vi "configUI.vi"() -> ()   [LabVIEW 2017, in "AppStateMachine editor node.lvclass"]
doc: "All child modules share this same UI. The UI allows for the configuration of Channels, Parameters, and Error Handling."
uses:
  AppStateMachine editor node.lvclass
  <vilib>/NI/Configuration Framework/Node/NodeRef.ctl
  <vilib>/NI/Configuration Framework/Node/NISE_CEF_Node.lvclass
  <vilib>/NI/AMC/Message Queue.ctl
  <vilib>/NI/AMC/Message.ctl
  <vilib>/NI/Tools/Keyed Array/KeyedArray.ctl
  <vilib>/NI/Configuration Framework/Node/UserEventRef.ctl
  <vilib>/NI/Configuration Framework/Controls/EventCluster.ctl
  <vilib>/NI/DCAF/Tag Editor Core/control module/configuration/error classification setting.ctl
  <vilib>/NI/Tag Bus Module Framework/runtime/error classification.ctl
  <vilib>/NI/Configuration Framework/Node/RefreshUIEvent.ctl
  <vilib>/NI/Configuration Framework/Node/CacheState.ctl
  <vilib>/NI/Configuration Framework/Node/StopEvent.ctl
  <vilib>/NI/Configuration Framework/Node/NodeChangeEvent.ctl
  <vilib>/NI/DCAF/Tag Editor Core/Table API/Available Tag Menu/channel action event.ctl
  <vilib>/NI/DCAF/Tag Editor Core/Table API/Available Tag Menu/dialog output action.ctl
  <vilib>/NI/Tag Bus Module Framework/channel/TBM channel.lvclass
  <vilib>/NI/Tag Bus/tag/tag descriptor.lvclass
  <vilib>/NI/DCAF/Tag Editor Core/Table API/Table Manager/Call Back Ref Type Def.ctl
  <vilib>/NI/DCAF/Tag Editor Core/Configuration Editor/Classes/Engine Parent/Engine Parent Editor Node.lvclass
  <vilib>/NI/DCAF/Tag Editor Core/Configuration Editor/Classes/Module editor node/module editor node.lvclass
  C:/Program Files (x86)/National Instruments/LabVIEW 2017/vi.lib/NI/Configuration Framework/serializable node/NISE_CEF_serializable node.lvclass
  <vilib>/NI/DCAF/Tag Editor Core/Table API/Table Manager/references.ctl
  <vilib>/NI/DCAF/Tag Editor Core/Table API/Table Manager/Menu Definition.ctl
  <vilib>/NI/DCAF/Tag Editor Core/Table API/Table Manager/Menu Options.ctl
  <vilib>/NI/DCAF/Tag Editor Core/control module/configuration/control module configuration.lvclass
  C:/Program Files (x86)/National Instruments/LabVIEW 2017/vi.lib/NI/Configuration Framework/serializable configuration/NISE_CEF_serializable configuration.lvclass
  module/configuration/AppStateMachine configuration.lvclass
  C:/Program Files (x86)/National Instruments/LabVIEW 2017/vi.lib/NI/DCAF/Tag Editor Core/control module/configuration/control module configuration.lvclass
  C:/Program Files (x86)/National Instruments/LabVIEW 2017/vi.lib/NI/Tag Bus Module Framework/module configuration/TBM module configuration.lvclass
  C:/Program Files (x86)/National Instruments/LabVIEW 2017/vi.lib/NI/DCAF/Tag Editor Core/control module/editor node/control module editor.lvclass
  C:/Program Files (x86)/National Instruments/LabVIEW 2017/vi.lib/NI/DCAF/Tag Editor Core/Configuration Editor/Classes/Module editor node/module editor node.lvclass
  module/configuration/AppStateMachine configuration.lvclass/AppStateMachine configuration.ctl
  <vilib>/NI/DCAF/Tag Editor Core/control module/configuration/control module configuration.lvclass/control module configuration.ctl
  <vilib>/NI/Configuration Framework/serializable configuration/NISE_CEF_serializable configuration.lvclass/NISE_CEF_serializable configuration.ctl
  <vilib>/NI/Tag Bus Module Framework/channel/channel classification.ctl
  module/configuration/Read PrechargeTimeout.vi
  module/configuration/Read SynchronizeTimeout.vi
  module/configuration/Read DCLinkSteadyStateTimeout.vi
  module/configuration/Read PrechargeLevel.vi
  module/configuration/Read DCLinkSteadyState.vi
  module/configuration/Write PrechargeTimeout.vi
  module/configuration/Write SynchronizeTimeout.vi
  module/configuration/Write DCLinkSteadyStateTimeout.vi
  module/configuration/Write PrechargeLevel.vi
  module/configuration/Write DCLinkSteadyState.vi
  <vilib>/NI/DCAF/Tag Editor Core/control module/configuration/Write error classifications.vi
  <vilib>/NI/Tag Bus Module Framework/module configuration/TBM module configuration.lvclass
  <vilib>/NI/DCAF/Tag Editor Core/Configuration Editor/Classes/Module editor node/Read Module Configuration.vi
  <vilib>/NI/DCAF/Tag Editor Core/control module/editor node/read fixed channel configuration.vi
  <vilib>/NI/DCAF/Tag Editor Core/Configuration Editor/Classes/Module editor node/Write Module Configuration.vi
  <vilib>/Utility/LVClass/Get LV Class Name.vi
  <vilib>/NI/Configuration Framework/error generator/NISE_error generator.vi
  <vilib>/NI/Configuration Framework/serializable configuration/NISE_CEF_serializable configuration.lvclass
  <vilib>/NI/DCAF/Tag Editor Core/Table API/Listbox/Multi Column Listbox.lvclass
  <vilib>/NI/Configuration Framework/NISE_CEF_TreeControl.lvlib
  <vilib>/NI/DCAF/Tag Editor Core/Table API/Table Manager.lvlib
  <vilib>/NI/DCAF UI Toolkit/Controls/DCAF UI Elements.lvlib
  <vilib>/NI/Tools/Keyed Array/Tools_KeyedArray.lvlib
  <vilib>/NI/AMC/AMC.lvlib
  <vilib>/NI/DCAF/Tag Editor Core/Table API/Table Manager/Table Manager.lvclass
  <vilib>/NI/DCAF/Tag Editor Core/control module/editor node/control module editor.lvclass
  <vilib>/NI/Tag Bus Module Framework/runtime/TBM module execution interface.lvclass
panel:
  in  "Enum":i32
  in  "user event out":refnum<user-event>
  in  "Top Level Tab Control":T1(tab)
  in  "DCLinkSteadyState":dbl caption="DCLink Steady State (V)"
  in  "PrechargeLevel":dbl caption="Precharge Level (V)"
  in  "DCLinkSteadyStateTimeout":u32 caption="DCLink Steady State Timeout (ms)"
  in  "SynchronizeTimeout":u32 caption="Synchronize Timeout (ms)"
  in  "PrechargeTimeout":u32 caption="Precharge Timeout (ms)"
  in  "Channels Listbox":i32(listbox)
  in  "mapall":bool
  in  "mapwriters":bool
  in  "Parameters Listbox":i32(listbox)
  in  "error classifications":T2[](array[typedef])
  in  "node change":T4
  in  "stop event":T5
  in  "cache state":T6
  in  "refresh UI":T7
  in  "user event":T8
  in  "main queue":T9
  in  "node ref":T10
  # "(Single-Click to Edit)"
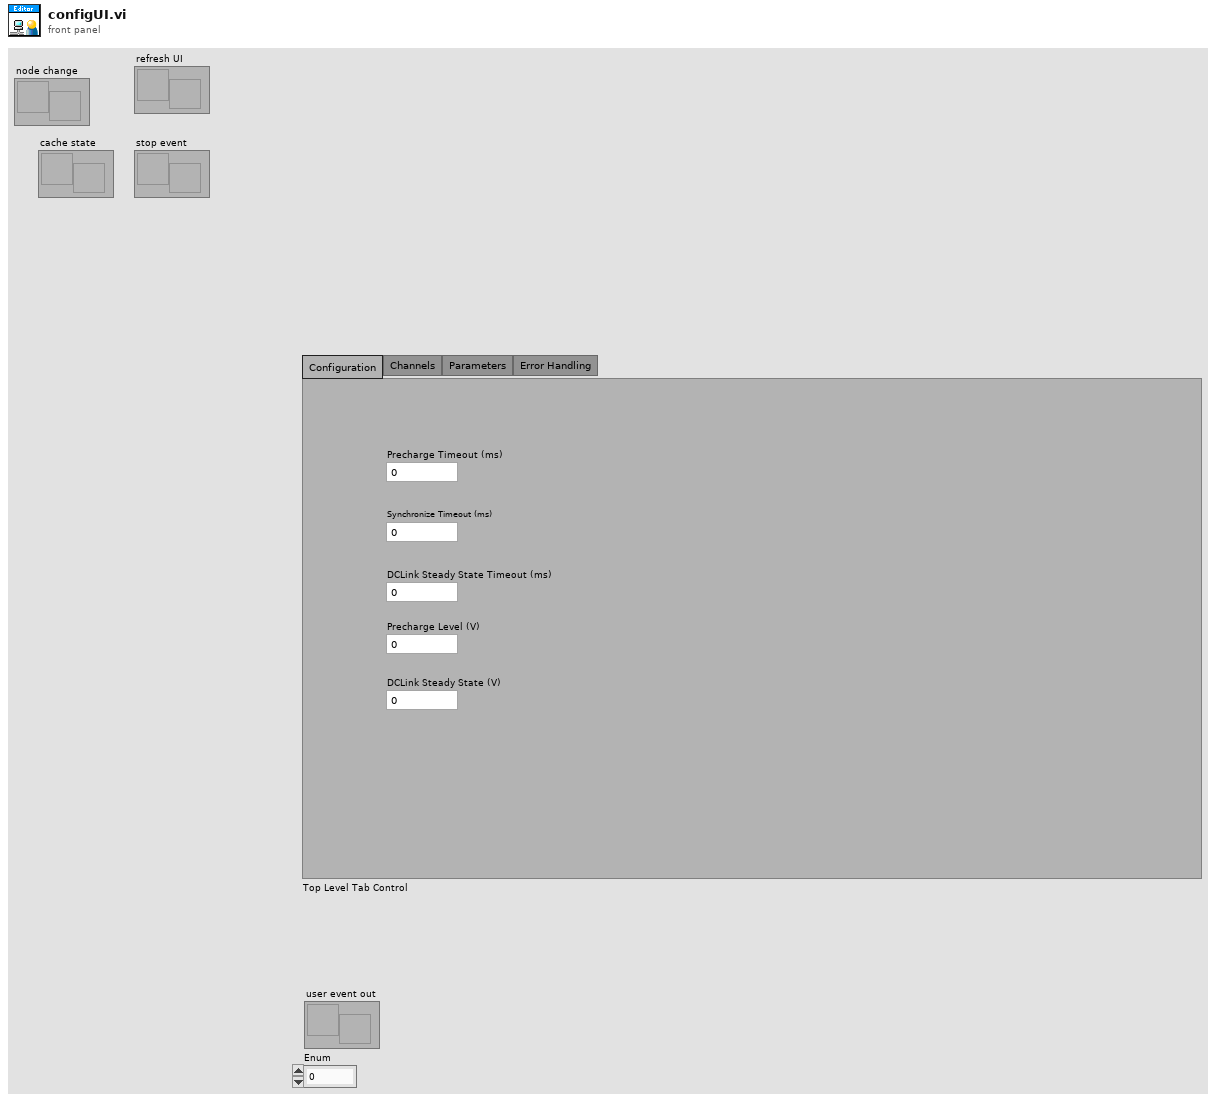
[diagram p1: front panel]
types:
  T1 = enum32{"Configuration", "Channels", "Parameters", "Error Handling"}
  T2 = typedef "control module configuration.lvclass/error classification setting.ctl" = cluster{"code":i32, "error classification":T3}
  T3 = typedef "TBM module execution interface.lvclass/error classification.ctl" = enum16{"unknown", "none", "trivial", "recoverable", "critical"}
  T4 = typedef "NISE_CEF_Node.lvclass/NodeChangeEvent.ctl" = refnum<user-event>
  T5 = typedef "NISE_CEF_Node.lvclass/StopEvent.ctl" = refnum<user-event>
  T6 = typedef "NISE_CEF_Node.lvclass/CacheState.ctl" = refnum<user-event>
  T7 = typedef "NISE_CEF_Node.lvclass/RefreshUIEvent.ctl" = refnum<user-event>
  T8 = typedef "NISE_CEF_Node.lvclass/UserEventRef.ctl" = refnum<user-event>
  T9 = typedef "AMC.lvlib/Message Queue.ctl" = refnum<queue>
  T10 = typedef "NISE_CEF_Node.lvclass/NodeRef.ctl" = refnum<data-value>
  T11 = typedef "Table Manager.lvlib/Table Manager.lvclass/Menu Definition.ctl" = cluster{"Menu Name":string, "Menu Options":T12}
  T12 = typedef "Table Manager.lvlib/Table Manager.lvclass/Menu Options.ctl" = enum16{"Always Show", "Show When Used", "Show When Empty"}
  T13 = typedef "Table Manager.lvlib/Table Manager.lvclass/references.ctl" = cluster{"stop event":T5, "refresh UI":T7, "cache state":T6, "node change":T4, "user event out":refnum<user-event>, "main queue":T9, "user event":T8}
  T14 = typedef "Table Manager.lvlib/Column.lvclass/Column Descriptor.ctl" = cluster{"name":string, "caption":string, "Column Type":T15, "Params":string, "AutoSizeMode":i32, "FillWeight":sgl, "MinWidth":u32, "tooltip":string, "Enum Reference":refnum<vi>, "Channel suffix":string, "Read Only":bool, "Call Back VI":T16, "DT Dependency":i32, "name dependency":i32, "data type":T17, "Custom Column":refnum<class "Column.lvclass">}
  T15 = typedef "Table Manager.lvlib/Column.lvclass/Column Type.ctl" = enum16{"String", "Mapping", "Enum", "Custom"}
  T16 = typedef "Table Manager.lvlib/Table Manager.lvclass/Call Back Ref Type Def.ctl" = refnum<vi>
  T17 = typedef "tag bus.lvlib/tag descriptor.lvclass/Data Type.ctl" = enum16{"Double", "Single", "I64", "I32", "I16", "I8", "U64", "U32", "U16", "U8", "Boolean", "String", "Array of Double", "Array of Single", "Array of I64", "Array of I32", "Array of I16", "Array of I8", "Array of U64", "Array of U32", "Array of U16", "Array of U8", "Array of Boolean", "Array of String"}
  T18 = typedef "Table Manager.lvlib/Table Manager.lvclass/object ref.ctl" = cluster{"engine":refnum<data-value>, "Node Ref":refnum<data-value>}
  T19 = typedef "Table Manager.lvlib/Table Manager.lvclass/Table Events.ctl" = cluster{"Menu Selection":refnum<user-event>}
  T20 = typedef "NISE_CEF_TreeControl.lvlib/EventCluster.ctl" = cluster{"command":string, "data":string}
  T21 = typedef "TBM channel.lvclass/channel classification.ctl" = enum16{"input data", "output data", "processing parameter", "processing result"}
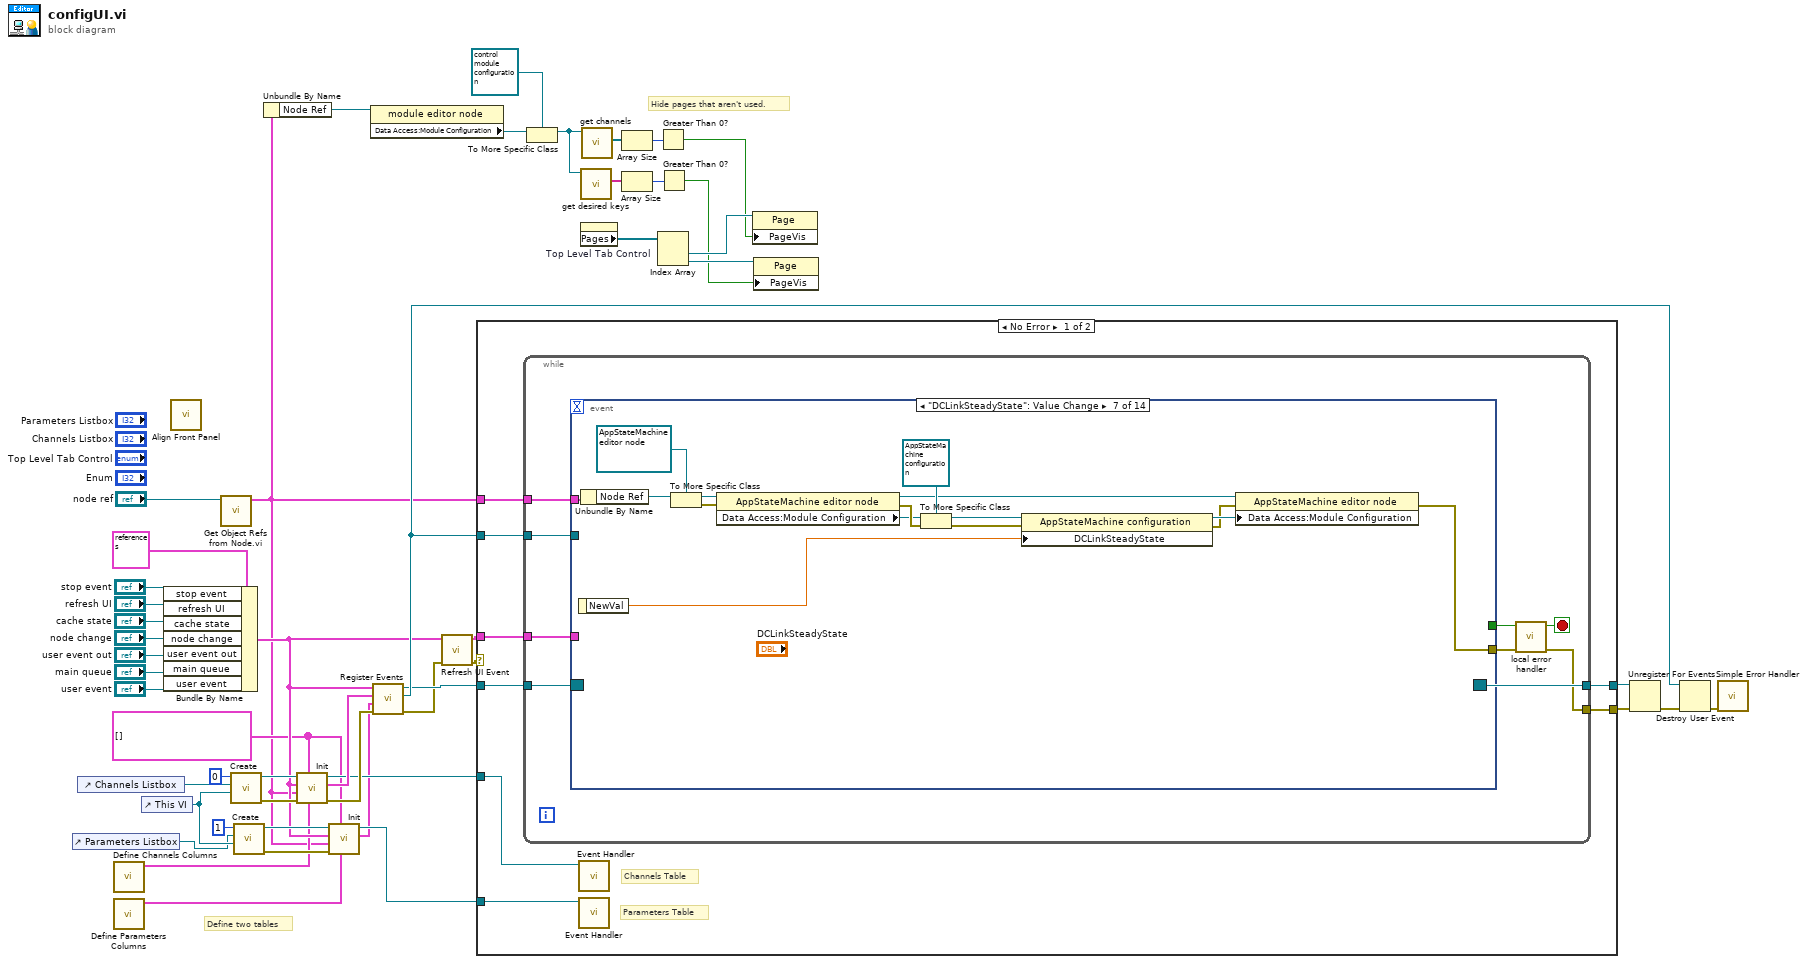
[diagram p0: block diagram]
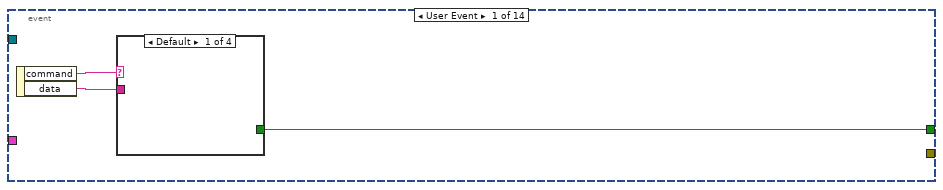
[diagram p2: hidden frame]
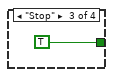
[diagram p4: hidden frame]
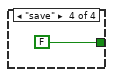
[diagram p5: hidden frame]
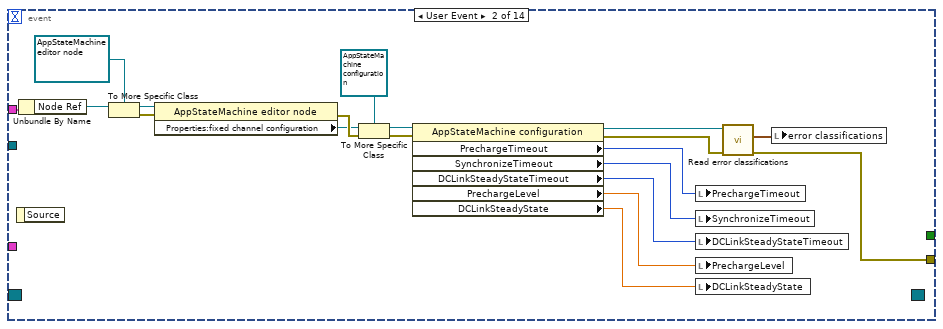
[diagram p6: hidden frame]
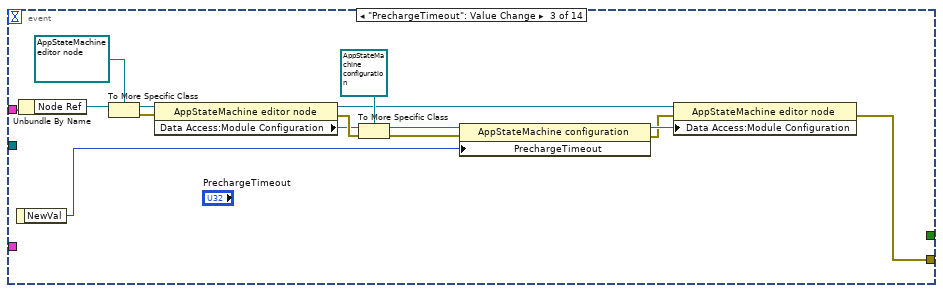
[diagram p7: hidden frame]
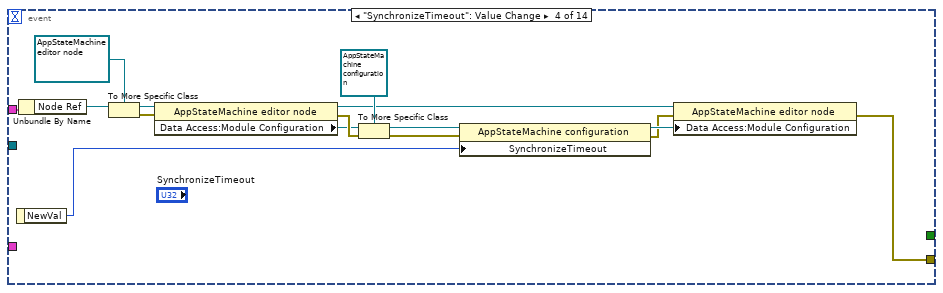
[diagram p8: hidden frame]
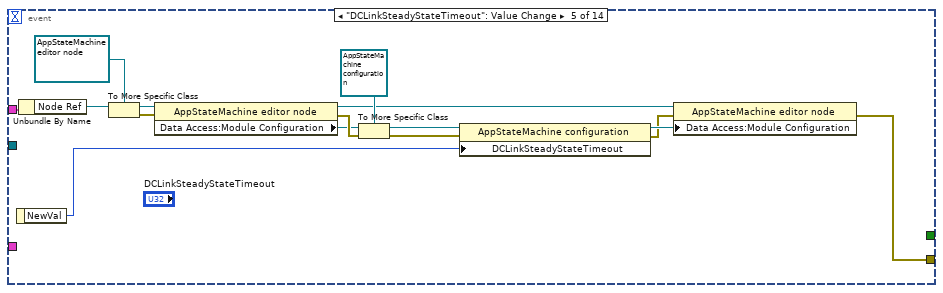
[diagram p9: hidden frame]
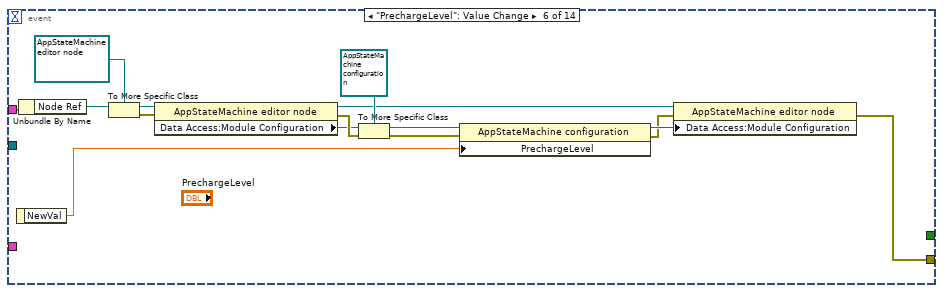
[diagram p10: hidden frame]
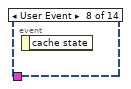
[diagram p11: hidden frame]
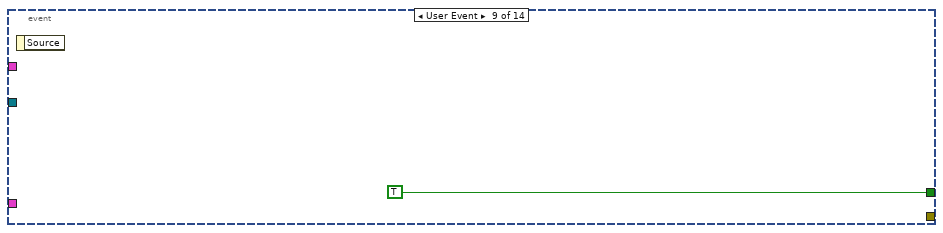
[diagram p12: hidden frame]
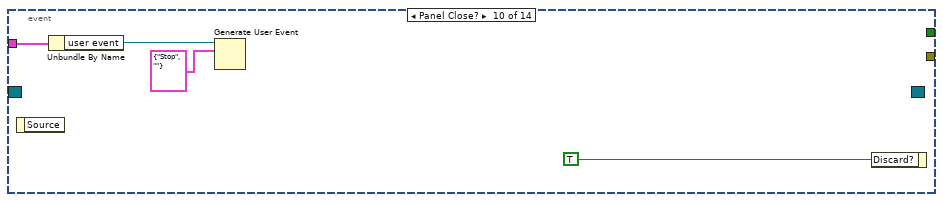
[diagram p13: hidden frame]
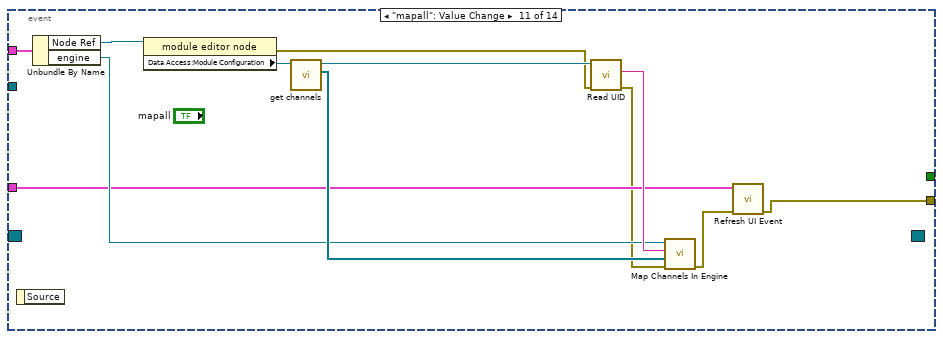
[diagram p14: hidden frame]
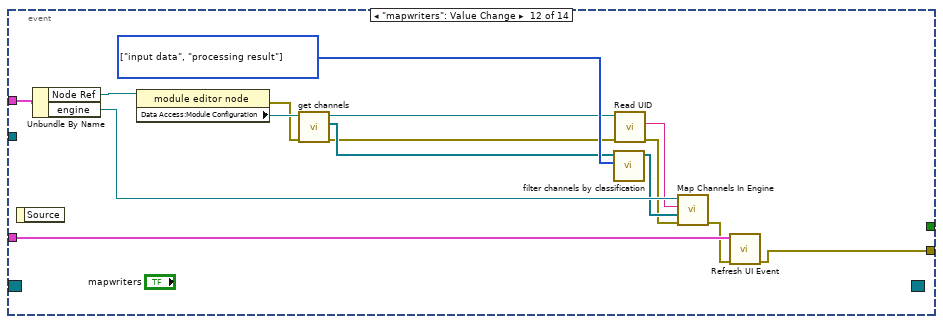
[diagram p15: hidden frame]
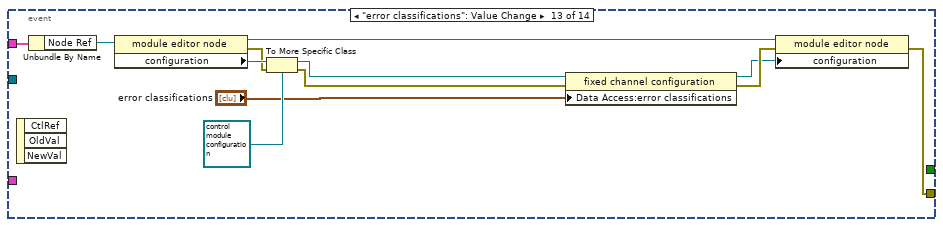
[diagram p16: hidden frame]
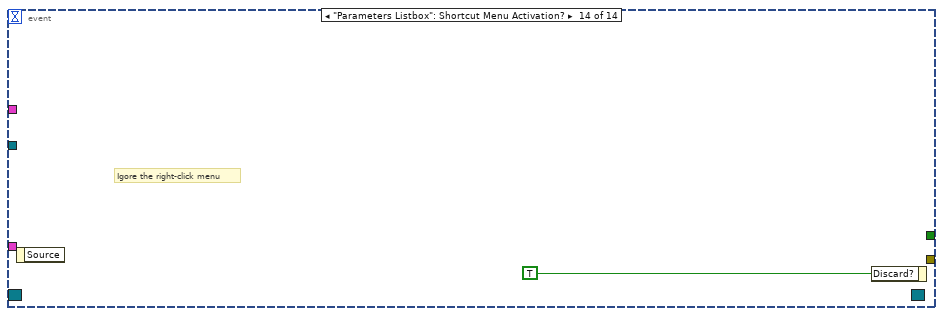
[diagram p17: hidden frame]
diagram:
  w15 = T11[] [] ("Right-Click Menu")
  # "Define two tables"
  # "Hide pages that aren't used."
  n1 = control-ref of="Parameters Listbox"() -> (w18:refnum<vi>)
  n2 = control-ref of="Channels Listbox"() -> (w26:refnum<vi>)
  n3 = call <vilib>:"Define Channels Columns.vi"() -> ("Column Descriptors"=w17:T14[])  [unwired: 11 in]
  n4 = call <vilib>:"Define Parameters Columns.vi"() -> ("Column Descriptors"=w16:T14[])  [unwired: 11 in]
  n5 = control-ref of="This VI"() -> (w22:refnum<vi>)
  n6 = Bundle By Name(cluster=T13 {"stop event"=refnum, "refresh UI"=refnum, "cache state"=refnum, "node change"=refnum, "user event out"=refnum, "main queue"=refnum, "user event"=refnum} ("Event References"), "stop event"="stop event", "refresh UI"="refresh UI", "cache state"="cache state", "node change"="node change", "user event out"="user event out", "main queue"="main queue", "user event"="user event") -> (w19:T13)
  n7 = call <vilib>:"Align Front Panel.vi"() -> ()  [unwired: 10 in, 2 out]
  n8 = call <vilib>:"Get Object Refs from Node.vi.vi"("node ref"="node ref") -> ("Node object refs"=w7:T18)  [unwired: 9 in, 1 out]
  n9 = call <vilib>:"Create.vi"("Top VI"=w22, "Listbox"=w26, "Index"=0) -> ("error out"=w29:errorcluster, "reference out"=w30:refnum<class "Multi Column Listbox.lvclass">)  [unwired: 7 in]
  n10 = call <vilib>:"Create.vi"("Top VI"=w22, "Listbox"=w18, "Index"=1) -> ("error out"=w25:errorcluster, "reference out"=w24:refnum<class "Multi Column Listbox.lvclass">)  [unwired: 7 in]
  n11 = Unbundle By Name(w7) -> ("Node Ref"=w5:refnum<data-value>)
  n12 = call-dynamic "Init.vi"("Column Descriptors"=w17, "Right-Click Menu"=w15, "error in (no error)"=w29, "Node object refs"=w7, "Event References"=w19, "Multi Column Listbox in"=w30) -> ("error out"=w28:errorcluster, "Table Events"=w40:T19, "Multi Column Listbox out"=w27:refnum<class "Multi Column Listbox.lvclass">)  [unwired: 3 in]
  n13 = call-dynamic "Init.vi"("Column Descriptors"=w16, "Right-Click Menu"=w15, "error in (no error)"=w25, "Node object refs"=w7, "Event References"=w19, "Multi Column Listbox in"=w24) -> ("Table Events"=w20:T19, "Multi Column Listbox out"=w21:refnum<class "Multi Column Listbox.lvclass">)  [unwired: 3 in, 1 out]
  n14 = property class="module editor node"(reference=w5) -> ("Data Access:Module Configuration"=w6:refnum<class "TBM module configuration.lvclass">)  [unwired: 1 in, 2 out]
  n15 = call <vilib>:"Register Events.vi"("error in (no error)"=w28, "Parameters Table Events"=w20, "Channels Table Events"=w40, "Event References"=w19) -> ("error out"=w33:errorcluster, "Channel Action"=w39:refnum<user-event>, "Event Registration Refnum"=w38:refnum<event-registration>)  [unwired: 5 in]
  n16 = call <vilib>:"Refresh UI Event.vi"("error in (no error)"=w33, "Event References"=w19) -> ("error out"=w34:errorcluster, "Event References out"=w32:T13)  [unwired: 8 in]
  n17 = case shown="No Error" w34 {
    selector: w34 -> [_ w212]
    tunnel: w38 -> [w58 w211]
    tunnel: [w57 w211] -> w50
    tunnel: [w55 w212] -> w49
    tunnel: w39 -> [w56 _]
    tunnel: w7 -> [w54 _]
    tunnel: w32 -> [w53 _]
    tunnel: w27 -> [w52 _]
    tunnel: w21 -> [w51 _]
    frame No Error {
      # "Parameters Table"
      # "Channels Table"
      n18 = while {
        tunnel: w58 -> [w67]
        tunnel: [w66] -> w57
        tunnel: w56 -> [w65]
        tunnel: [w61] -> w55
        tunnel: w54 -> [w60]
        tunnel: w53 -> [w59]
        stop <- w63 stop-if-true
        n19 = event shown="[6] \"DCLinkSteadyState\": Value Change" {
          selector: w67 -> [_ _ _ _ _ _ _ _ _ _ _ _ _ _]
          dyn-events: [_ _ _ _ _ _ _ _ _ _ _ _ _ _] -> w66
          timeout: _ -> [_ _ _ _ _ _ _ _ _ _ _ _ _ _]
          tunnel: [w70 _ _ _ _ _ _ _ TRUE _ _ _ _ _] -> w64
          tunnel: [_ w89 w94 w109 w124 w139 w154 _ _ _ w177 w193 w209 _] -> w62
          tunnel: w65 -> [_ _ _ _ _ _ _ _ _ _ _ _ _ _]
          tunnel: w60 -> [_ w91 w106 w121 w136 w151 w166 _ _ _ w181 w194 w208 _]
          tunnel: w59 -> [_ _ _ _ _ _ _ _ _ w169 w176 w192 _ _]
          event User Event {
            n20 = event-data() -> ("command"=w69:string, "data"=w68:string)  [unwired: 1 in]
            n21 = case shown="Default" w69 {
              tunnel: [_ _ TRUE FALSE] -> w70
              tunnel: w68 -> [_ _ _ _]
              frame Default {
              }
              frame "Refresh" {
              }
              frame "Stop" {
              }
              frame "save" {
              }
            }
          }
          event User Event {
            n22 = event-data() -> ()  [unwired: 1 in, 1 out]
            n23 = Unbundle By Name(w91) -> ("Node Ref"=w90:refnum<data-value>)
            n24 = To More Specific Class(target class=refnum<data-value> refnum ("data value reference"), reference=w90) -> (specific class reference=w88:refnum<data-value>, error out=w85:errorcluster)  [unwired: 1 in]
            n25 = property class="AppStateMachine editor node"(reference=w88, error in=w85) -> (error out=w86:errorcluster, "Properties:fixed channel configuration"=w84:refnum<class "control module configuration.lvclass">)  [unwired: 1 out]
            n26 = To More Specific Class(target class=refnum<class "AppStateMachine configuration.lvclass"> refnum ("AppStateMachine configuration"), reference=w84, error in=w86) -> (specific class reference=w83:refnum<class "AppStateMachine configuration.lvclass">, error out=w82:errorcluster)
            n27 = property class="AppStateMachine configuration"(reference=w83, error in=w82) -> (reference out=w81:refnum<class "AppStateMachine configuration.lvclass">, error out=w80:errorcluster, "PrechargeTimeout"=w77:u32, "SynchronizeTimeout"=w76:u32, "DCLinkSteadyStateTimeout"=w75:u32, "PrechargeLevel"=w74:dbl, "DCLinkSteadyState"=w73:dbl)
            n28 = local write "PrechargeTimeout"(w77) -> ()
            n29 = local write "SynchronizeTimeout"(w76) -> ()
            n30 = local write "DCLinkSteadyStateTimeout"(w75) -> ()
            n31 = local write "PrechargeLevel"(w74) -> ()
            n32 = local write "DCLinkSteadyState"(w73) -> ()
            n33 = call <vilib>:"Read error classifications.vi"("error in"=w80, "control module configuration in"=w81) -> ("error out"=w89:errorcluster, "error classifications"=w87:T2[])  [unwired: 7 in, 1 out]
            n34 = local write "error classifications"(w87) -> ()
          }
          event "PrechargeTimeout": Value Change {
            n35 = event-data() -> ("NewVal"=w96:u32)  [unwired: 1 in]
            n36 = Unbundle By Name(w106) -> ("Node Ref"=w105:refnum<data-value>)
            n37 = To More Specific Class(target class=refnum<data-value> refnum ("data value reference"), reference=w105) -> (specific class reference=w104:refnum<data-value>, error out=w102:errorcluster)  [unwired: 1 in]
            n38 = property class="AppStateMachine editor node"(reference=w104, error in=w102) -> (reference out=w95:refnum<data-value>, error out=w103:errorcluster, "Data Access:Module Configuration"=w101:refnum<class "TBM module configuration.lvclass">)
            n39 = To More Specific Class(target class=refnum<class "AppStateMachine configuration.lvclass"> refnum ("AppStateMachine configuration"), reference=w101, error in=w103) -> (specific class reference=w100:refnum<class "AppStateMachine configuration.lvclass">, error out=w99:errorcluster)
            n40 = property class="AppStateMachine configuration"(reference=w100, error in=w99, "PrechargeTimeout"=w96) -> (reference out=w93:refnum<class "AppStateMachine configuration.lvclass">, error out=w92:errorcluster)
            n41 = property class="AppStateMachine editor node"(reference=w95, error in=w92, "Data Access:Module Configuration"=w93) -> (error out=w94:errorcluster)  [unwired: 1 out]
          }
          event "SynchronizeTimeout": Value Change {
            n42 = event-data() -> ("NewVal"=w111:u32)  [unwired: 1 in]
            n43 = Unbundle By Name(w121) -> ("Node Ref"=w120:refnum<data-value>)
            n44 = To More Specific Class(target class=refnum<data-value> refnum ("data value reference"), reference=w120) -> (specific class reference=w119:refnum<data-value>, error out=w117:errorcluster)  [unwired: 1 in]
            n45 = property class="AppStateMachine editor node"(reference=w119, error in=w117) -> (reference out=w110:refnum<data-value>, error out=w118:errorcluster, "Data Access:Module Configuration"=w116:refnum<class "TBM module configuration.lvclass">)
            n46 = To More Specific Class(target class=refnum<class "AppStateMachine configuration.lvclass"> refnum ("AppStateMachine configuration"), reference=w116, error in=w118) -> (specific class reference=w115:refnum<class "AppStateMachine configuration.lvclass">, error out=w114:errorcluster)
            n47 = property class="AppStateMachine configuration"(reference=w115, error in=w114, "SynchronizeTimeout"=w111) -> (reference out=w108:refnum<class "AppStateMachine configuration.lvclass">, error out=w107:errorcluster)
            n48 = property class="AppStateMachine editor node"(reference=w110, error in=w107, "Data Access:Module Configuration"=w108) -> (error out=w109:errorcluster)  [unwired: 1 out]
          }
          event "DCLinkSteadyStateTimeout": Value Change {
            n49 = event-data() -> ("NewVal"=w126:u32)  [unwired: 1 in]
            n50 = Unbundle By Name(w136) -> ("Node Ref"=w135:refnum<data-value>)
            n51 = To More Specific Class(target class=refnum<data-value> refnum ("data value reference"), reference=w135) -> (specific class reference=w134:refnum<data-value>, error out=w132:errorcluster)  [unwired: 1 in]
            n52 = property class="AppStateMachine editor node"(reference=w134, error in=w132) -> (reference out=w125:refnum<data-value>, error out=w133:errorcluster, "Data Access:Module Configuration"=w131:refnum<class "TBM module configuration.lvclass">)
            n53 = To More Specific Class(target class=refnum<class "AppStateMachine configuration.lvclass"> refnum ("AppStateMachine configuration"), reference=w131, error in=w133) -> (specific class reference=w130:refnum<class "AppStateMachine configuration.lvclass">, error out=w129:errorcluster)
            n54 = property class="AppStateMachine configuration"(reference=w130, error in=w129, "DCLinkSteadyStateTimeout"=w126) -> (reference out=w123:refnum<class "AppStateMachine configuration.lvclass">, error out=w122:errorcluster)
            n55 = property class="AppStateMachine editor node"(reference=w125, error in=w122, "Data Access:Module Configuration"=w123) -> (error out=w124:errorcluster)  [unwired: 1 out]
          }
          event "PrechargeLevel": Value Change {
            n56 = event-data() -> ("NewVal"=w141:dbl)  [unwired: 1 in]
            n57 = Unbundle By Name(w151) -> ("Node Ref"=w150:refnum<data-value>)
            n58 = To More Specific Class(target class=refnum<data-value> refnum ("data value reference"), reference=w150) -> (specific class reference=w149:refnum<data-value>, error out=w147:errorcluster)  [unwired: 1 in]
            n59 = property class="AppStateMachine editor node"(reference=w149, error in=w147) -> (reference out=w140:refnum<data-value>, error out=w148:errorcluster, "Data Access:Module Configuration"=w146:refnum<class "TBM module configuration.lvclass">)
            n60 = To More Specific Class(target class=refnum<class "AppStateMachine configuration.lvclass"> refnum ("AppStateMachine configuration"), reference=w146, error in=w148) -> (specific class reference=w145:refnum<class "AppStateMachine configuration.lvclass">, error out=w144:errorcluster)
            n61 = property class="AppStateMachine configuration"(reference=w145, error in=w144, "PrechargeLevel"=w141) -> (reference out=w138:refnum<class "AppStateMachine configuration.lvclass">, error out=w137:errorcluster)
            n62 = property class="AppStateMachine editor node"(reference=w140, error in=w137, "Data Access:Module Configuration"=w138) -> (error out=w139:errorcluster)  [unwired: 1 out]
          }
          event "DCLinkSteadyState": Value Change {
            n63 = event-data() -> ("NewVal"=w156:dbl)  [unwired: 1 in]
            n64 = Unbundle By Name(w166) -> ("Node Ref"=w165:refnum<data-value>)
            n65 = To More Specific Class(target class=refnum<data-value> refnum ("data value reference"), reference=w165) -> (specific class reference=w164:refnum<data-value>, error out=w162:errorcluster)  [unwired: 1 in]
            n66 = property class="AppStateMachine editor node"(reference=w164, error in=w162) -> (reference out=w155:refnum<data-value>, error out=w163:errorcluster, "Data Access:Module Configuration"=w161:refnum<class "TBM module configuration.lvclass">)
            n67 = To More Specific Class(target class=refnum<class "AppStateMachine configuration.lvclass"> refnum ("AppStateMachine configuration"), reference=w161, error in=w163) -> (specific class reference=w160:refnum<class "AppStateMachine configuration.lvclass">, error out=w159:errorcluster)
            n68 = property class="AppStateMachine configuration"(reference=w160, error in=w159, "DCLinkSteadyState"=w156) -> (reference out=w153:refnum<class "AppStateMachine configuration.lvclass">, error out=w152:errorcluster)
            n69 = property class="AppStateMachine editor node"(reference=w155, error in=w152, "Data Access:Module Configuration"=w153) -> (error out=w154:errorcluster)  [unwired: 1 out]
          }
          event User Event {
            n70 = event-data() -> ()  [unwired: 1 in, 1 out]
          }
          event User Event {
            n71 = event-data() -> ()  [unwired: 1 in, 1 out]
          }
          event Panel Close? {
            n72 = event-data() -> ()  [unwired: 1 in, 1 out]
            n73 = Unbundle By Name(w169) -> ("user event"=w168:T8)
            n74 = Generate User Event(user event=w168, event data cluster=T20 {"command"="Stop", "data"=""} ("event data")) -> ()  [unwired: 2 in, 2 out]
            n75 = event-data("Discard?"=TRUE) -> ()  [unwired: 1 in, 1 out]
          }
          event "mapall": Value Change {
            n76 = event-data() -> ()  [unwired: 1 in, 1 out]
            n77 = Unbundle By Name(w181) -> ("Node Ref"=w180:refnum<data-value>, "engine"=w179:refnum<data-value>)
            n78 = property class="module editor node"(reference=w180) -> (error out=w173:errorcluster, "Data Access:Module Configuration"=w175:refnum<class "TBM module configuration.lvclass">)  [unwired: 1 in, 1 out]
            n79 = call-dynamic "get channels.vi"("module configuration in"=w175) -> ("channels"=w183:refnum<class "TBM channel.lvclass">[], "module configuration out"=w174:refnum<class "TBM module configuration.lvclass">)  [unwired: 9 in]
            n80 = call <vilib>:"Read UID.vi"("error in"=w173, "configuration in"=w174) -> ("error out"=w172:errorcluster, "instance id"=w182:string)  [unwired: 7 in, 1 out]
            n81 = call <vilib>:"Map Channels In Engine.vi"("error in (no error)"=w172, "channels"=w183, "instance id"=w182, "Engine DVR"=w179) -> ("error out"=w178:errorcluster)  [unwired: 7 in]
            n82 = call <vilib>:"Refresh UI Event.vi"("error in (no error)"=w178, "Event References"=w176) -> ("error out"=w177:errorcluster)  [unwired: 8 in, 1 out]
          }
          event "mapwriters": Value Change {
            w197 = T21[] [enum."input data", enum."processing result"] items=["input data", "output data", "processing parameter", "processing result"] ("allowed classifications")
            n83 = event-data() -> ()  [unwired: 1 in, 1 out]
            n84 = Unbundle By Name(w194) -> ("Node Ref"=w195:refnum<data-value>, "engine"=w191:refnum<data-value>)
            n85 = property class="module editor node"(reference=w195) -> (error out=w184:errorcluster, "Data Access:Module Configuration"=w186:refnum<class "TBM module configuration.lvclass">)  [unwired: 1 in, 1 out]
            n86 = call-dynamic "get channels.vi"("module configuration in"=w186) -> ("channels"=w196:refnum<class "TBM channel.lvclass">[], "module configuration out"=w185:refnum<class "TBM module configuration.lvclass">)  [unwired: 9 in]
            n87 = call <vilib>:"filter channels by classification.vi"("allowed classifications"=w197, "channels in"=w196) -> ("channels out"=w189:refnum<class "TBM channel.lvclass">[])  [unwired: 9 in]
            n88 = call <vilib>:"Read UID.vi"("error in"=w184, "configuration in"=w185) -> ("error out"=w188:errorcluster, "instance id"=w190:string)  [unwired: 7 in, 1 out]
            n89 = call <vilib>:"Map Channels In Engine.vi"("error in (no error)"=w188, "channels"=w189, "instance id"=w190, "Engine DVR"=w191) -> ("error out"=w187:errorcluster)  [unwired: 7 in]
            n90 = call <vilib>:"Refresh UI Event.vi"("error in (no error)"=w187, "Event References"=w192) -> ("error out"=w193:errorcluster)  [unwired: 8 in, 1 out]
          }
          event "error classifications": Value Change {
            n91 = event-data() -> ()  [unwired: 1 in, 3 out]
            n92 = Unbundle By Name(w208) -> ("Node Ref"=w203:refnum<data-value>)
            n93 = property class="module editor node"(reference=w203) -> (reference out=w207:refnum<data-value>, error out=w199:errorcluster, "configuration"=w202:refnum<class "NISE_CEF_serializable configuration.lvclass">)  [unwired: 1 in]
            n94 = To More Specific Class(target class=refnum<class "control module configuration.lvclass"> refnum ("fixed channel configuration"), reference=w202, error in=w199) -> (specific class reference=w204:refnum<class "control module configuration.lvclass">, error out=w198:errorcluster)
            n95 = property class="fixed channel configuration"(reference=w204, error in=w198, "Data Access:error classifications"="error classifications") -> (reference out=w205:refnum<class "control module configuration.lvclass">, error out=w206:errorcluster)
            n96 = property class="module editor node"(reference=w207, error in=w206, "configuration"=w205) -> (error out=w209:errorcluster)  [unwired: 1 out]
          }
          event "Parameters Listbox": Shortcut Menu Activation? {
            # "Igore the right-click menu"
            n97 = event-data() -> ()  [unwired: 1 in, 1 out]
            n98 = event-data("Discard?"=TRUE) -> ()  [unwired: 1 in, 1 out]
          }
        }
        n99 = call <vilib>:"local error handler.vi"("error in (no error)"=w62, "Stop in"=w64) -> ("error out"=w61:errorcluster, "Stop out"=w63:bool)  [unwired: 8 in]
      }
      n100 = call-dynamic "Event Handler.vi"("Listbox in"=w52) -> ()  [unwired: 9 in, 2 out]
      n101 = call-dynamic "Event Handler.vi"("Listbox in"=w51) -> ()  [unwired: 9 in, 2 out]
    }
    frame Error {
    }
  }
  n102 = To More Specific Class(target class=refnum<class "control module configuration.lvclass"> refnum ("fixed channel configuration"), reference=w6) -> (specific class reference=w3:refnum<class "control module configuration.lvclass">)  [unwired: 1 in, 1 out]
  n103 = call-dynamic "get desired keys.vi"("fixed channel configuration in"=w3) -> ("desired keys"=w11:string[])  [unwired: 8 in, 2 out]
  n104 = property on="Top Level Tab Control" class="TabCtl (strict)"() -> ("Pages"=w8:refnum<vi>[])  [unwired: 2 in, 2 out]
  n105 = call-dynamic "get channels.vi"("fixed channel configuration in"=w3) -> ("channels"=w14:refnum<class "TBM channel.lvclass">[])  [unwired: 9 in, 1 out]
  n106 = Array Size(array=w14) -> (size(s)=w13:i32)
  n107 = Array Size(array=w11) -> (size(s)=w12:i32)
  n108 = Greater Than 0?(x=w13) -> (x > 0?=w2:bool)
  n109 = Index Array(array=w8) -> (element #1=w9:refnum<vi>, element #2=w10:refnum<vi>)  [unwired: 2 in]
  n110 = Greater Than 0?(x=w12) -> (x > 0?=w1:bool)
  n111 = property class="Page"(reference=w9, "PageVis"=w2) -> ()  [unwired: 1 in, 2 out]
  n112 = property class="Page"(reference=w10, "PageVis"=w1) -> ()  [unwired: 1 in, 2 out]
  n113 = Unregister For Events(event registration refnum=w50, error in=w49) -> (error out=w48:errorcluster)
  n114 = Destroy User Event(user event=w39, error in=w48) -> (error out=w47:errorcluster)
  n115 = call <vilib>:"Simple Error Handler.vi"("error in (no error)"=w47) -> ()  [unwired: 4 in, 5 out]
